vi "FTW-Request-Construct.vi"(5 "Server Address":string, 11 "error in":errorcluster) -> (4 "FTW-Request Out":refnum<class "FTW-Request.lvclass">, 15 "error out":errorcluster)   [LabVIEW 2013, in "FTW-Request.lvclass"]
uses:
  FTW-Request.lvclass
  Ether/FTW-Ether-EndpointType.ctl
  Endpoint/FTW-Endpoint.lvclass
  FTW-Request.lvclass/FTW-Request.ctl
  Ether/FTW-Ether.lvclass
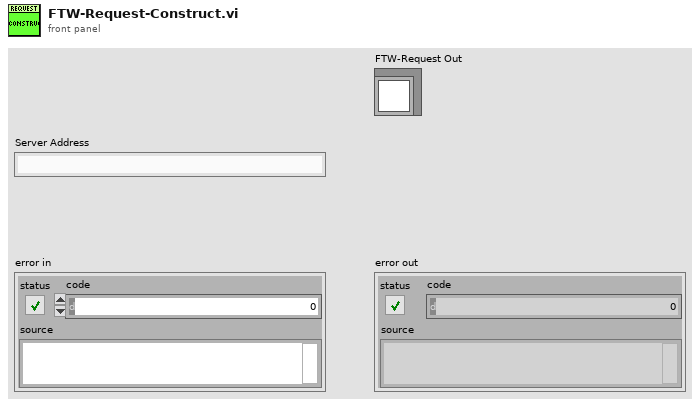
[diagram p1: front panel]
types:
  T1 = typedef "FTW-Ether.lvclass/FTW-Ether-EndpointType.ctl" = enum16{"Server", "Client", "Publisher", "Subscriber"}
  T2 = typedef "FTW-Ether.lvclass/FTW-Ether-MessageTransportScheme.ctl" = enum16{"In process (inproc://)", "TCP (tcp://)"}
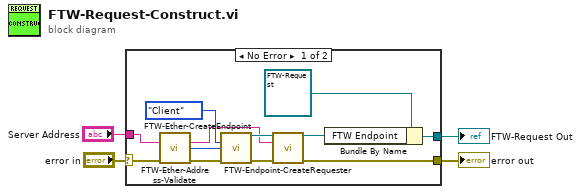
[diagram p0: block diagram]
diagram:
  n1 = case shown="No Error" "error in" {
    selector: "error in" -> [w15 w17]
    tunnel: [w8 w17] -> w2
    tunnel: [w16 _] -> w4
    tunnel: "Server Address" -> [w12 _]
    frame No Error {
      n2 = call "FTW-Ether-Address-Validate.vi"("Address"=w12, "error in"=w15) -> ("Sanitized Address"=w9:string, "Message Transport Scheme"=w7:T2, "error out"=w14:errorcluster)  [unwired: 11 in]
      n3 = call "FTW-Ether-CreateEndpoint.vi"("Endpoint Type"=FTW-Ether-EndpointType."Client", "Message Transport Scheme"=w7, "error in"=w14) -> ("FTW Endpoint"=w10:refnum<class "FTW-Endpoint.lvclass">, "error out"=w11:errorcluster)  [unwired: 11 in]
      n4 = call-dynamic "FTW-Endpoint-CreateRequester.vi"("FTW Endpoint"=w10, "Endpoint Address"=w9, "error in"=w11) -> ("FTW Endpoint out"=w5:refnum<class "FTW-Endpoint.lvclass">, "error out"=w8:errorcluster)  [unwired: 11 in]
      n5 = Bundle By Name(cluster=refnum<class "FTW-Request.lvclass"> refnum ("LVmsg_Client in"), "FTW Endpoint"=w5) -> (w16:refnum<class "FTW-Request.lvclass">)
    }
    frame Error {
    }
  }
  "FTW-Request Out" <- w4
  "error out" <- w2
